vi "SetWindowPosition.vi"(4 "y":i32, 6 "x":i32, 8 "No Error":errorcluster, 9 "Center y":bool, 10 "Center x":bool, 11 "Window [SDL_Window *]":i64 format="%.0x") -> (0 "Error Out":errorcluster)   [LabVIEW 2026, in "SDL3.lvlib" / "Video.lvlib"]
doc: "<B>Summary</B>\nRequest that the window's position be set.\n\n<B>Thread Safety</B>\nIf the window is in an exclusive fullscreen or maximized state, this request has no effect.\n\nThis can be used to reposition fullscreen-desktop windows onto a different display, however, as exclusive fullscreen windows are locked to a specific display, they can only be repositioned programmatically via <B>SDL_SetWindowFullscreenMode()</B>.\n\nOn some windowing systems this request is asynchronous and the new coordinates may not have have been applied immediately upon the return of this function. If an immediate change is required, call <B>SDL_SyncWindow()</B> to block until the changes have taken effect.\n\nWhen the window position changes, an <B>SDL_EVENT_WINDOW_MOVED</B> event will be emitted with the window's new coordinates. Note that the new coordinates may not match the exact coordinates requested, as some windowing systems can restrict the position of the window in certain scenarios (e.g. constraining the position so the window is always within desktop bounds). Additionally, as this is just a request, it can be denied by the windowing system."
uses:
  Video.lvlib
  <vilib>/Utility/error.llb/Error Cluster From Error Code.vi
  Error/Error.lvlib
  Lib/SDL3.dll
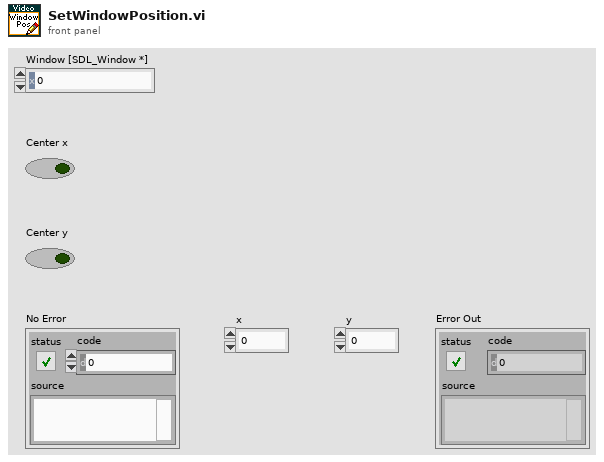
[diagram p1: front panel]
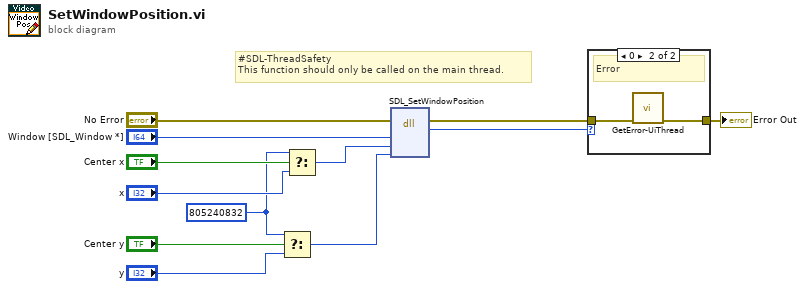
[diagram p0: block diagram]
diagram:
  w1 = 805240832 ("t")
  # "#SDL-ThreadSafety\nThis function should only be called on the main thread."
  n1 = Select(t=w1, s="Center y", f="y") -> (s? t:f=w3:i32)
  n2 = Select(t=w1, s="Center x", f="x") -> (s? t:f=w5:i32)
  n3 = dll-call lib="C:/Users/saukko/Dev/LV-SDL3/Sources/SDL3/Lib/SDL3.*" fn="SDL_SetWindowPosition"(error in="No Error", "window"="Window [SDL_Window *]", "x"=w5, "y"=w3) -> (error out=w9:errorcluster, "return type"=w8:i32)  [unwired: 5 in, 1 out]
  n4 = case shown="0" w8 {
    tunnel: w9 -> [w13 w15]
    tunnel: [w13 w14] -> w11
    frame Default {
      # "Ok"
    }
    frame 0 {
      # "Error"
      n5 = call "GetError-UiThread.vi"("No Error"=w15) -> ("error out"=w14:errorcluster)  [unwired: 10 in]
    }
  }
  "Error Out" <- w11
